vi "Prompt User for Init Type.vi"(8 "error in (no error)":errorcluster) -> (0 "error out":errorcluster, 2 "Create Limit Channels? out":bool, 3 "Path out":path)   [LabVIEW 2019, in "Profile Interpolation System Explorer.lvlib"]
uses:
  Profile Interpolation System Explorer.lvlib
panel:
  in  "Create Limit Channels?":bool
  in  "New Instance?":bool
  in  "OK":bool
  in  "Path":path
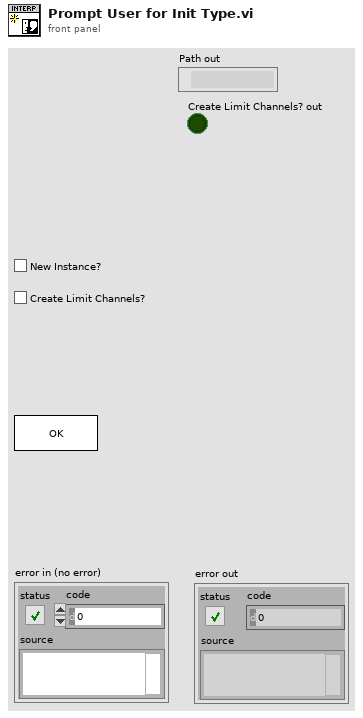
[diagram p1: front panel]
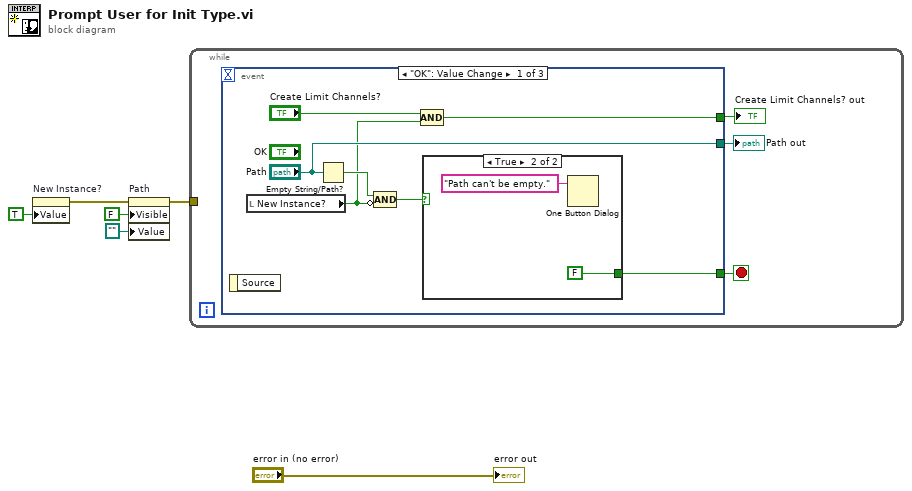
[diagram p0: block diagram]
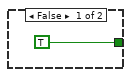
[diagram p2: hidden frame]
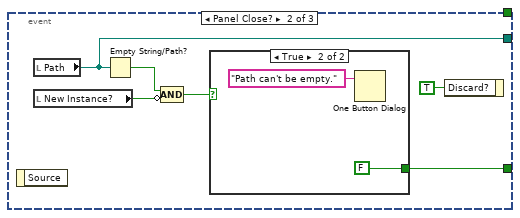
[diagram p3: hidden frame]
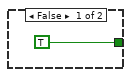
[diagram p4: hidden frame]
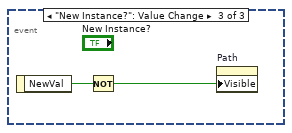
[diagram p5: hidden frame]
diagram:
  n1 = property on="New Instance?" class="Bool (strict)"("Value"=TRUE ("New Instance?")) -> (error out=w3:errorcluster)  [unwired: 2 in, 1 out]
  n2 = property on="Path" class="Path"(error in=w3, "Visible"=FALSE, "Value"=path "") -> (error out=w5:errorcluster)  [unwired: 1 in, 1 out]
  n3 = while {
    tunnel: w5 -> [_]
    stop <- w9 stop-if-true
    n4 = event shown="[0] \"OK\": Value Change" {
      selector: _ -> [_ _ _]
      dyn-events: _ -> [_ _ _]
      timeout: _ -> [_ _ _]
      tunnel: [w16 w25 _] -> w9
      tunnel: ["Path" w20 _] -> w8
      tunnel: [w10 _ _] -> w7
      event "OK": Value Change {
        n5 = event-data() -> ()  [unwired: 1 in, 1 out]
        n6 = local read "New Instance?"() -> (w11:bool)
        n7 = Empty String/Path?(string/path="Path") -> (empty?=w14:bool)
        n8 = Compound Arithmetic op=AND(w14, invert w11) -> (w13:bool)
        n9 = Compound Arithmetic op=AND("Create Limit Channels?", w11) -> (w10:bool)
        n10 = case shown="True" w13 {
          tunnel: [TRUE FALSE] -> w16
          frame False {
          }
          frame True {
            n11 = One Button Dialog(message="Path can't be empty.") -> ()  [unwired: 1 in, 1 out]
          }
        }
      }
      event Panel Close? {
        n12 = event-data() -> ()  [unwired: 1 in, 1 out]
        n13 = local read "Path"() -> (w20:path)
        n14 = local read "New Instance?"() -> (w24:bool)
        n15 = Empty String/Path?(string/path=w20) -> (empty?=w23:bool)
        n16 = Compound Arithmetic op=AND(w23, invert w24) -> (w22:bool)
        n17 = case shown="True" w22 {
          tunnel: [TRUE FALSE] -> w25
          frame False {
          }
          frame True {
            n18 = One Button Dialog(message="Path can't be empty.") -> ()  [unwired: 1 in, 1 out]
          }
        }
        n19 = event-data("Discard?"=TRUE) -> ()  [unwired: 1 in, 1 out]
      }
      event "New Instance?": Value Change {
        n20 = event-data() -> ("NewVal"=w30:bool)  [unwired: 1 in]
        n21 = Not(x=w30) -> (.not. x?=w29:bool)
        n22 = property on="Path" class="Path"("Visible"=w29) -> ()  [unwired: 2 in, 2 out]
      }
    }
    "Path out" <- w8
    "Create Limit Channels? out" <- w7
  }
  "error out" <- "error in (no error)"
